vi "dfd_Bundle Lattice Coef Cluster.vi"(8 "error in (no error)":errorcluster, 11 "filter coef":T1) -> (0 "error out":errorcluster, 3 "lattice coef":T3)   [LabVIEW 2017, in "NI_DigFilterLicensed.lvlib"]
uses:
  <vilib>/addons/Digital Filter Design/NI_DigFilterLicensed.lvlib
  <vilib>/addons/Digital Filter Design/_Objects.llb/DFD Filter Structure Type Selector.ctl
  <vilib>/addons/Digital Filter Design/_Objects.llb/DFD Filter Coef.ctl
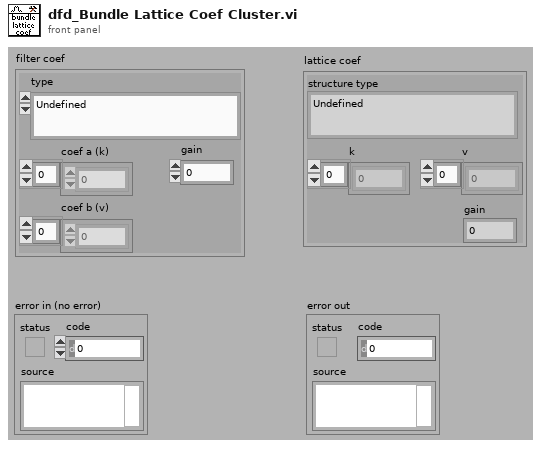
[diagram p1: front panel]
types:
  T1 = typedef "NI_DigFilterLicensed.lvlib/DFD Filter Coef.ctl" = cluster{"type":T2, "gain":dbl, "coef a (k)":dbl[], "coef b (v)":dbl[]}
  T2 = typedef "NI_DigFilterLicensed.lvlib/DFD Filter Structure Type Selector.ctl" = enum16{"Undefined", "FIR Direct Form", "FIR Direct Form Transposed", "FIR Symmetric", "FIR Antisymmetric", "IIR Direct Form I", "IIR Direct Form I Transposed", "IIR Direct Form II", "IIR Direct Form II Transposed", "IIR Cascaded Second Order Sections Form I", "IIR Cascaded Second Order Sections Form I Transposed", "IIR Cascaded Second Order Sections Form II", "IIR Cascaded Second Order Sections Form II Transposed", "Lattice Allpass (basic sections)", "Lattice Allpass (one multiplier sections)", "Lattice Allpass (normalized sections)", "Lattice AR (basic sections)", "Lattice AR (one multiplier sections)", "Lattice AR (normalized sections)", "Lattice MA (minimum phase)", "Lattice MA (maximum phase)", "Lattice ARMA (basic sections)", "Lattice ARMA (one multiplier sections)", "Lattice ARMA (normalized sections)"}
  T3 = cluster{"structure type":T2, "k":dbl[], "v":dbl[], "gain":dbl}
  T4 = enum16{"Undefined", "Basic", "One Multiplier", "Normalized"}
  T5 = typedef "NI_DigFilterLicensed.lvlib/DFD Lattice Type.ctl" = enum16{"Undefined", "Lattice Allpass", "Lattice AR", "Lattice MA (min)", "Lattice MA (max)", "Lattice ARMA"}
  T6 = cluster{"type":T2, "k [M~1]":dbl[], "coef b (v)":dbl[], "gain":dbl}
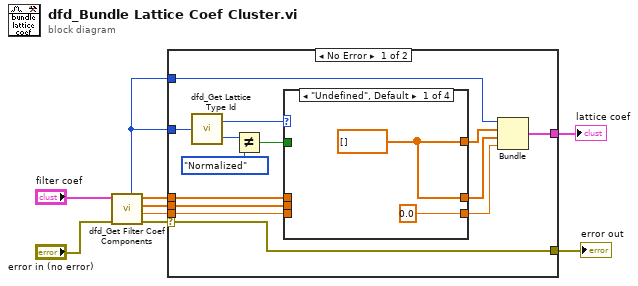
[diagram p0: block diagram]
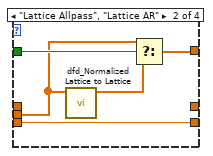
[diagram p2: hidden frame]
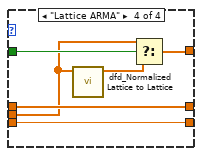
[diagram p4: hidden frame]
diagram:
  n1 = call <vilib>:"dfd_Get Filter Coef Components.vi"("error in (no error)"="error in (no error)", "filter coef"="filter coef") -> ("error out"=w3:errorcluster, "gain"=w8:dbl, "coef a (k)"=w7:dbl[], "coef b (v)"=w6:dbl[], "type"=w1:T2)  [unwired: 5 out]
  n2 = case shown="No Error" w3 {
    selector: w3 -> [w11 w39]
    tunnel: [w23 _] -> w9
    tunnel: w8 -> [w16 _]
    tunnel: w7 -> [w15 _]
    tunnel: w6 -> [w14 _]
    tunnel: w1 -> [w12 _]
    tunnel: [w11 w39] -> w2
    tunnel: w1 -> [w10 _]
    frame No Error {
      n3 = call <vilib>:"dfd_Get Lattice Type Id.vi"("structure type"=w12) -> ("lattice type"=w13:T5, "section type"=w18:T4)
      n4 = Not Equal?(x=w18, y=T4."Normalized" ("section type")) -> (x != y?=w17:bool)
      n5 = case shown="\"Undefined\", Default" w13 {
        tunnel: w14 -> [_ _ _ w38]
        tunnel: w15 -> [_ w28 w31 w33]
        tunnel: w16 -> [_ w30 w32 w37]
        tunnel: [w24 w26 w31 w35] -> w20
        tunnel: [w24 _ _ w38] -> w21
        tunnel: [0.0 ("gain") w30 w32 w37] -> w22
        tunnel: w17 -> [_ w29 _ w36]
        frame "Undefined", Default {
          w24 = dbl[] [] ("coef a (k)")
        }
        frame "Lattice Allpass", "Lattice AR" {
          n6 = call <vilib>:"dfd_Normalized Lattice to Lattice.vi"("k & ^k"=w28) -> ("k [M~1]"=w27:dbl[])  [unwired: 10 out]
          n7 = Select(t=w28, s=w29, f=w27) -> (s? t:f=w26:dbl[])
        }
        frame "Lattice MA (min)", "Lattice MA (max)" {
        }
        frame "Lattice ARMA" {
          n8 = call <vilib>:"dfd_Normalized Lattice to Lattice.vi"("k & ^k"=w33) -> ("k [M~1]"=w34:dbl[])  [unwired: 10 out]
          n9 = Select(t=w33, s=w36, f=w34) -> (s? t:f=w35:dbl[])
        }
      }
      n10 = Bundle("type"=w10, "k [M~1]"=w20, "coef b (v)"=w21, "gain"=w22) -> (w23:T6)  [unwired: 1 out]
    }
    frame Error {
    }
  }
  "error out" <- w2
  "lattice coef" <- w9
